vi "Cam Area.vi"() -> ()   [LabVIEW 2016]
panel:
  out "Cam Area":dbl
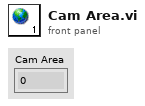
[diagram p1: front panel]
diagram:
